vi "例6-13.vi"() -> ()   [LabVIEW 2019]
uses:
  <vilib>/Analysis/NI_AALPro.lvlib
  <vilib>/measure/NI_MABase.lvlib
panel:
  in  "采样点数":dbl=100.0
  in  "采样频率":dbl=100.0
  in  "信号频率":dbl=10.0
  out "自功率谱波形":T1(graph)
  out "信号波形":waveform(dbl)(graph)
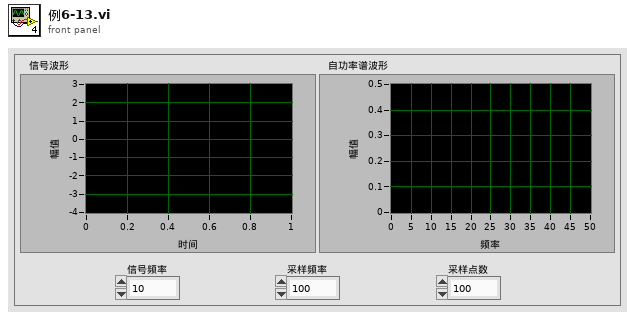
[diagram p1: front panel]
types:
  T1 = cluster{i32, "df":dbl, "Power Spectrum (V^2 rms)":dbl[]}
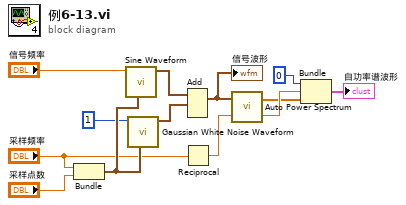
[diagram p0: block diagram]
diagram:
  n1 = Bundle("采样频率"="采样频率", "采样点数"="采样点数") -> (w12:cluster{"采样频率":dbl, "采样点数":dbl})  [unwired: 1 in]
  n2 = call <vilib>:"Sine Waveform.vi"("sampling info"=w12, "frequency"="信号频率") -> ("signal out"=w9:waveform(dbl))  [unwired: 8 in, 1 out]
  n3 = call <vilib>:"Gaussian White Noise Waveform.vi"("sampling info"=w12, "standard deviation"=1) -> ("signal out"=w8:waveform(dbl))  [unwired: 8 in, 1 out]
  n4 = Add(1:w8, 2:w9) -> (0:w7:waveform(dbl))  [unwired: 1 in, 1 out]
  "信号波形" <- w7
  n5 = Reciprocal(x="采样频率") -> (1/x=w5:dbl)
  n6 = call <vilib>:"Auto Power Spectrum.vi"("dt"=w5, "Signal (V)"=w7) -> ("df"=w3:dbl, "Power Spectrum (V^2 rms)"=w2:dbl[])
  n7 = Bundle(0, "df"=w3, "Power Spectrum (V^2 rms)"=w2) -> (→"自功率谱波形":T1)  [unwired: 1 in]
